vi "Slack-Spawn Subpanel Dialog.vi"(0 "SubPanel":refnum<vi>, 5 "Defaults":path, 7 "client_id":string, 9 "client_secret":string) -> (8 "close event":refnum<user-event>)   [LabVIEW 2015]
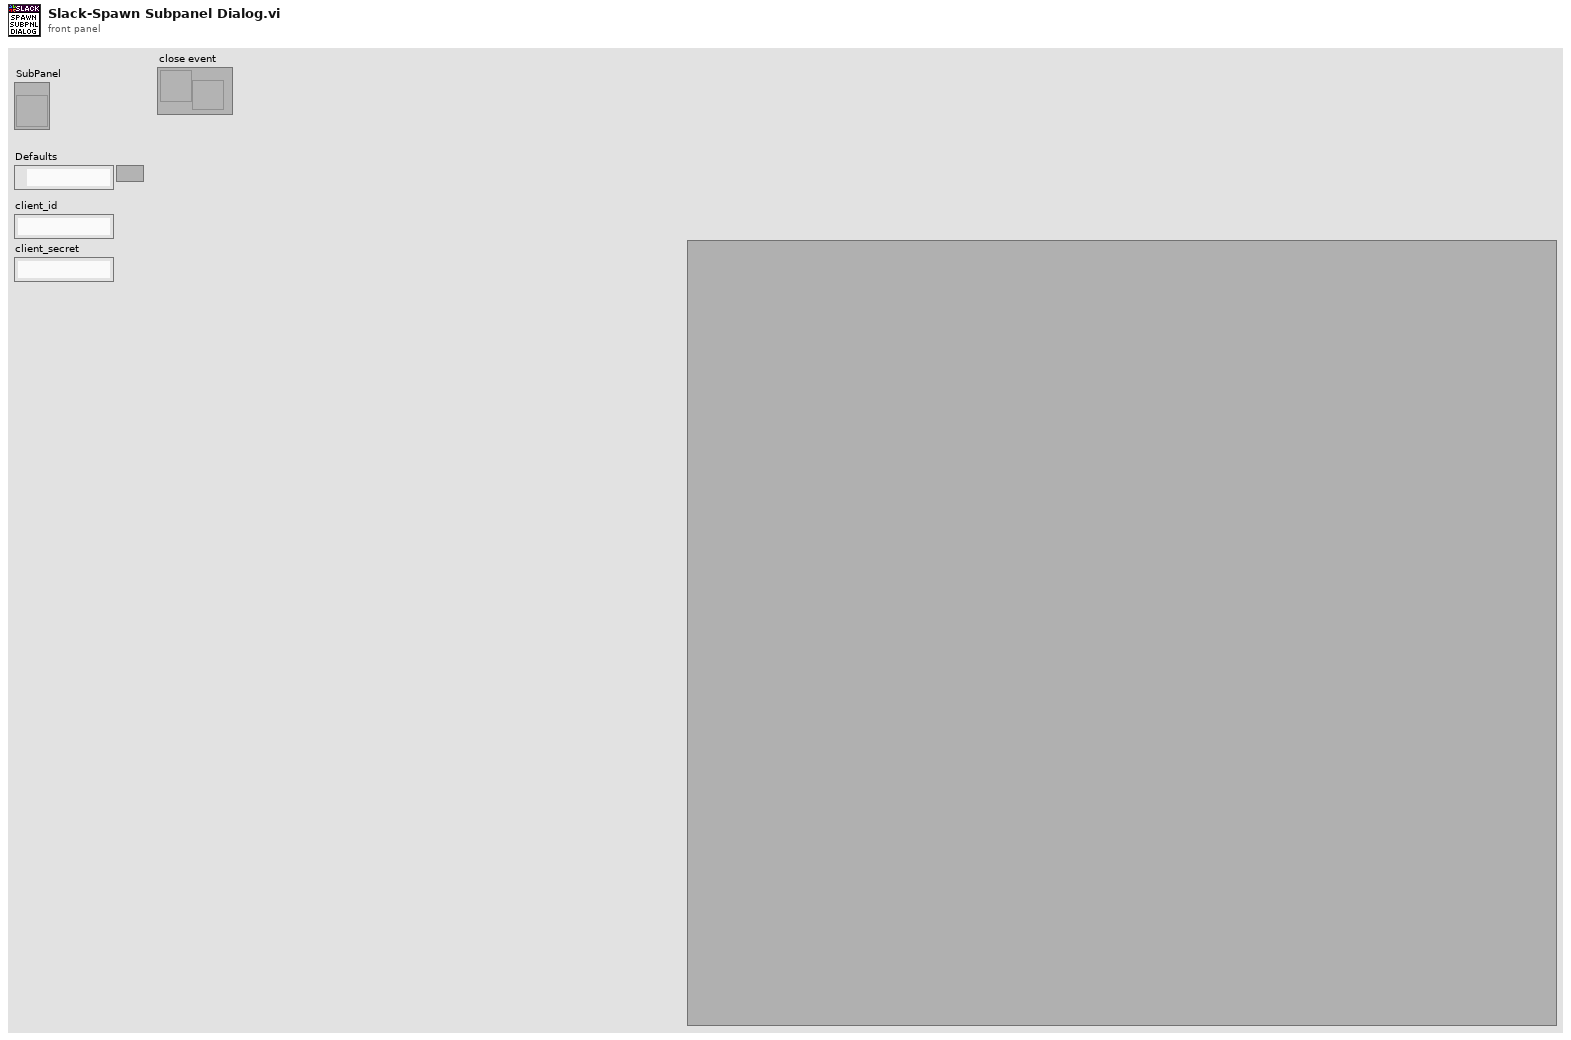
[diagram p1: front panel]
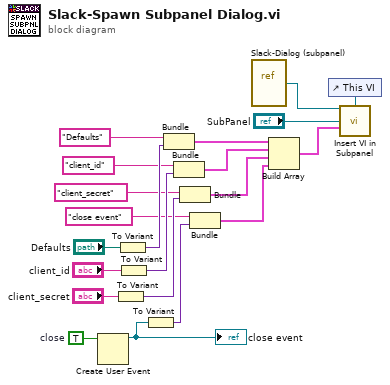
[diagram p0: block diagram]
diagram:
  w5 = TRUE  # close
  n1 = Create User Event(user event datatype=w5) -> (user event=w4:refnum<user-event>)  [unwired: 1 in, 1 out]
  "close event" <- w4
  n2 = To Variant(anything="client_secret") -> (Variant=w11:variant)
  n3 = To Variant(anything="Defaults") -> (Variant=w16:variant)
  n4 = To Variant(anything="client_id") -> (Variant=w15:variant)
  n5 = To Variant(anything=w4) -> (Variant=w3:variant)
  n6 = Bundle("Defaults", "Variant"=w16) -> (w9:cluster{string, "Variant":variant})  [unwired: 1 in]
  n7 = Bundle("client_id", "Variant"=w15) -> (w8:cluster{string, "Variant":variant})  [unwired: 1 in]
  n8 = Bundle("client_secret", "Variant"=w11) -> (w7:cluster{string, "Variant":variant})  [unwired: 1 in]
  n9 = Bundle("close event", "Variant"=w3) -> (w1:cluster{string, "Variant":variant})  [unwired: 1 in]
  n10 = vi-ref "Slack-Dialog (subpanel).vi"() -> (w21:refnum<vi>)
  n11 = Build Array(w9, w8, w7, w1) -> (w6:cluster{string, "Variant":variant}[])
  n12 = control-ref of="This VI"() -> (w20:refnum<vi>)
  n13 = call "Insert VI in Subpanel.vi"("VI Ref"=w21, "Parent"=w20, "SubPanel"="SubPanel", "inputs"=w6) -> ()  [unwired: 10 in, 2 out]
